vi "LinakUtilities.vi"(5 "LinakUtil":T1, 7 "Linak Address":u8=1, 8 "error in (no error)":errorcluster, 10 "Request(mm)":dbl=20.0 min=0.0 max=100000.0 step=10.0) -> (0 "error out":errorcluster, 1 "Target(mm)":dbl, 2 "AbsPosition":dbl, 3 "ThereYet?":bool)   [LabVIEW 2021]
uses:
  LINAKUTIL.ctl
  Registers.ctl
  <vilib>/Plasmionique/MB Master/MB_Master_TCP/MB_Master_TCP.lvclass
  Applications/National Instruments/LabVIEW 2021 64-bit/vi.lib/Plasmionique/MB Master/MB_Master/MB_Master.lvclass
  CPPSW/Systems/Cross-System/Fetch+RampsGlobal.vi
  <vilib>/Plasmionique/MB Master/MB Master.lvlib
  Applications/National Instruments/LabVIEW 2021 64-bit/vi.lib/Plasmionique/MB Master/MB_Master_TCP/MB_Master_TCP.lvclass
panel:
  in  "LINAK Gateway IP Address":string
  in  "Timeout (ms)":i32=500
  out "Request(pulses)":u16
  out "Target(pulses)":u16
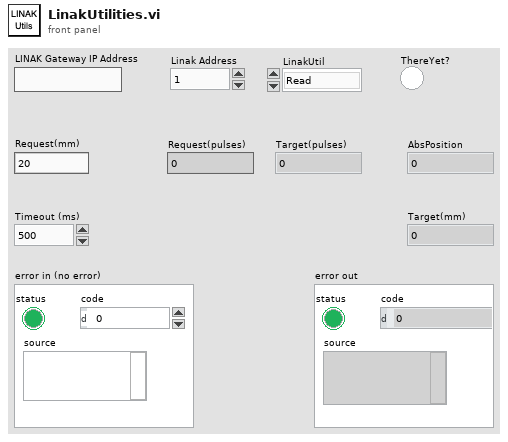
[diagram p1: front panel]
types:
  T1 = typedef "LINAKUTIL.ctl" = enum16{"Read", "ReadTarget", "WriteTarget", "SingleGo", "GlobalGo", "SafetySet", "WriteReadGo", "STOP"}
  T2 = typedef "Registers.ctl" = enum16{"Null", "TargetPosition", "Move"}
  T3 = typedef "LINAKStatusCluster.ctl" = cluster{"RunStatus":enum16{"Idle", "RunningOut", "RunningIn", "WaitingToRun", "InitOut", "InitIn"}, "ActualPosition(pulses)":u16, "DistanceFromTarget(pulses)":u16, "Status1":string, "ReasonForLastStop":string, "SupplyVoltage(V)":dbl, "Current(A)":dbl, "InternalTemp(C)":i16, "FETtemp(C)":i16}
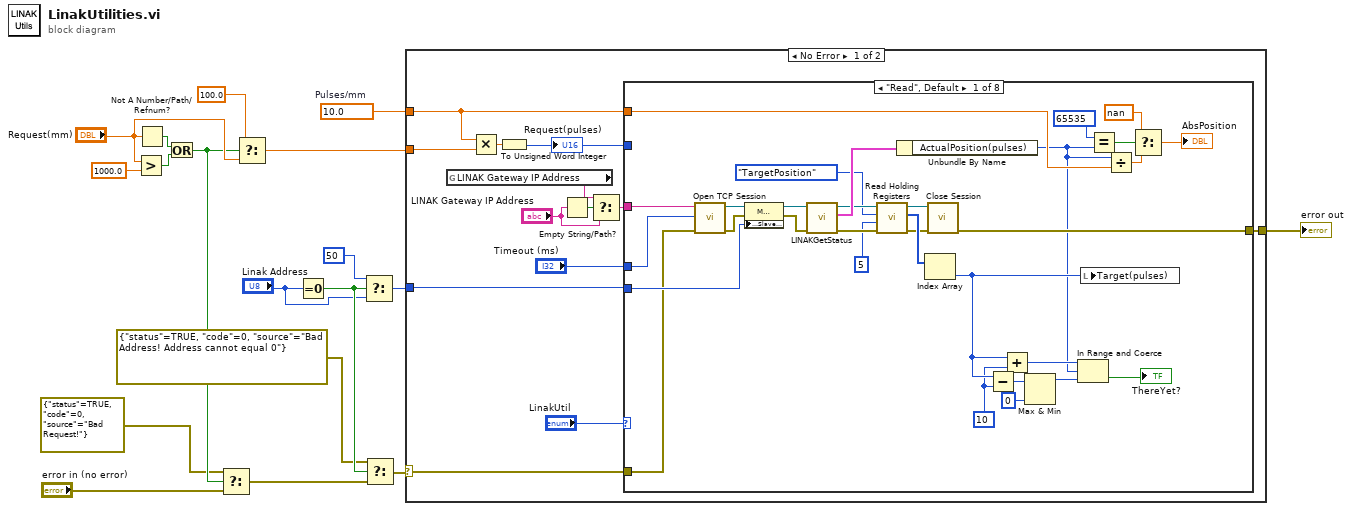
[diagram p0: block diagram]
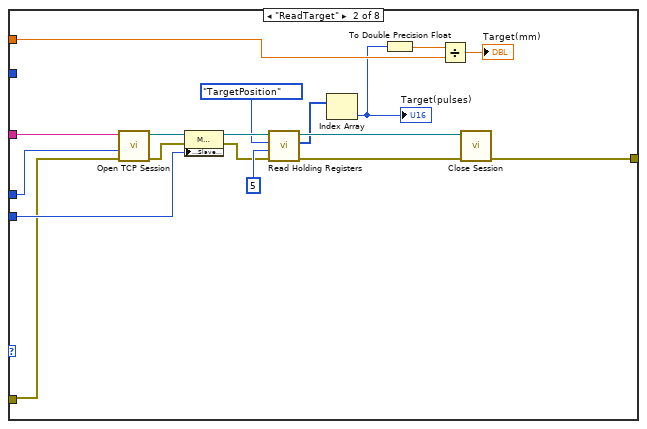
[diagram p2: hidden frame]
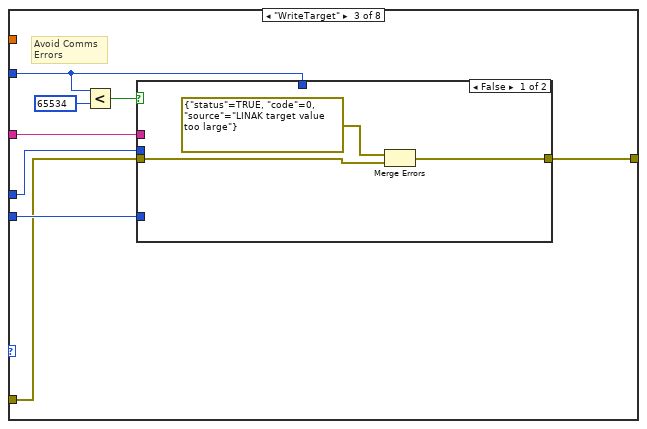
[diagram p3: hidden frame]
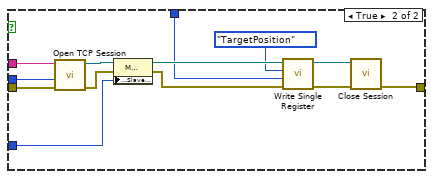
[diagram p4: hidden frame]
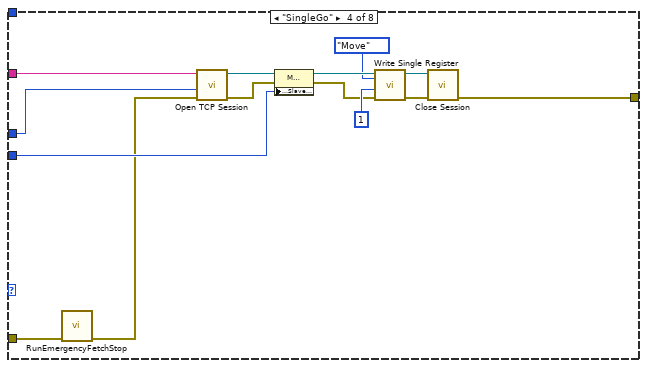
[diagram p5: hidden frame]
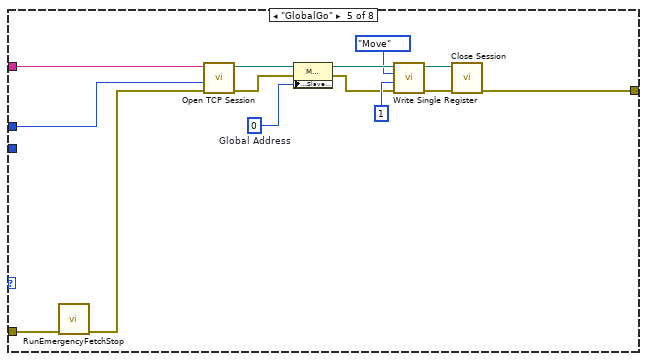
[diagram p6: hidden frame]
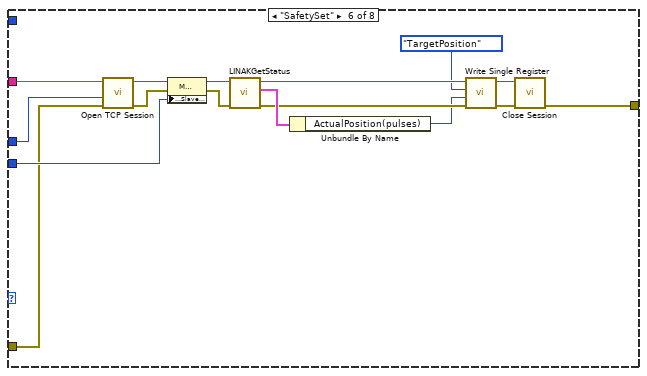
[diagram p7: hidden frame]
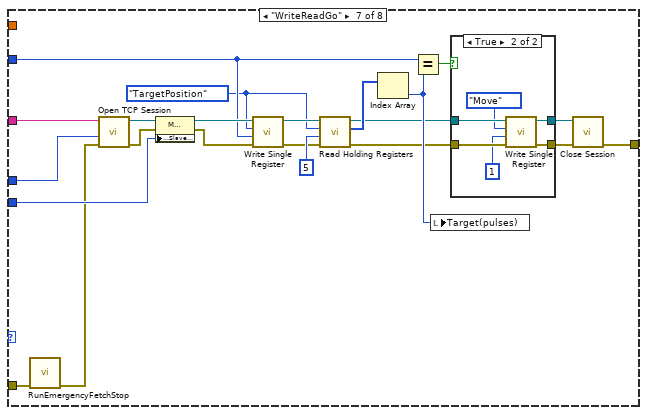
[diagram p8: hidden frame]
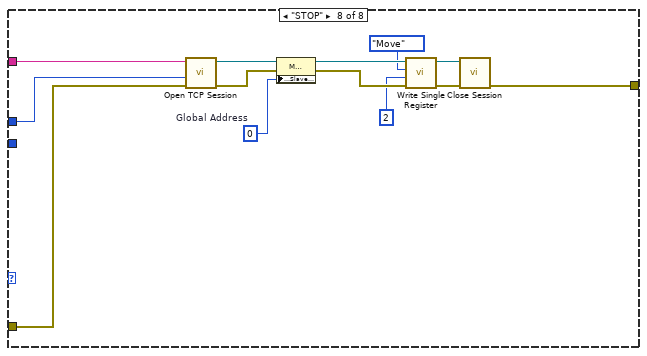
[diagram p10: hidden frame]
diagram:
  w1 = 10.0  # Pulses/mm
  n1 = Greater?(x="Request(mm)", y=1000.0) -> (0:w14:bool)
  n2 = Not A Number/Path/Refnum?(number/path/refnum="Request(mm)") -> (NaN/Path/Refnum?=w15:bool)
  n3 = Or(x=w15, y=w14) -> (x .or. y?=w9:bool)
  n4 = Select(t=errorcluster {"status"=TRUE, "code"=0, "source"="Bad Request!"}, s=w9, f="error in (no error)") -> (s? t:f=w6:errorcluster)
  n5 = Select(t=100.0, s=w9, f="Request(mm)") -> (s? t:f=w12:dbl)
  n6 = Equal To 0?(x="Linak Address") -> (x = 0?=w7:bool)
  n7 = Select(t=u8 50, s=w7, f="Linak Address") -> (s? t:f=w16:u8)
  n8 = Select(t=errorcluster {"status"=TRUE, "code"=0, "source"="Bad Address! Address cannot equal 0"}, s=w7, f=w6) -> (s? t:f=w4:errorcluster)
  n9 = case shown="No Error" w4 {
    selector: w4 -> [w20 w192]
    tunnel: [w28 w192] -> w18
    tunnel: w16 -> [w27 _]
    tunnel: w12 -> [w26 _]
    tunnel: w1 -> [w19 _]
    frame No Error {
      n10 = global read "Fetch+RampsGlobal.vi" "LINAK Gateway IP Address"() -> (w22:string)
      n11 = Multiply(x=w19, y=w26) -> (x*y=w31:dbl)
      n12 = To Unsigned Word Integer(number=w31) -> (unsigned 16bit integer=w30:u16)
      "Request(pulses)" <- w30
      n13 = Empty String/Path?(string/path="LINAK Gateway IP Address") -> (empty?=w24:bool)
      n14 = Select(t=w22, s=w24, f="LINAK Gateway IP Address") -> (s? t:f=w21:string)
      n15 = case shown="\"Read\", Default" "LinakUtil" {
        tunnel: w30 -> [_ _ w82 _ _ _ w161 _]
        tunnel: w19 -> [w61 w79 _ _ _ _ _ _]
        tunnel: w27 -> [w60 w80 w88 w118 _ w145 w170 _]
        tunnel: "Timeout (ms)" -> [w52 w73 w86 w116 w131 w143 w166 w184]
        tunnel: w21 -> [w51 w74 w87 w117 w132 w144 w167 w185]
        tunnel: w20 -> [w48 w72 w85 w106 w119 w142 w150 w183]
        tunnel: [w40 w65 w84 w115 w130 w135 w151 w190] -> w28
        frame "Read", Default {
          w53 = u16 10 ("y")
          n16 = call <vilib>:"Open TCP Session.vi"("error in (no error)"=w48, "Timeout (10000)"=w52, "IP Address"=w51) -> ("error out"=w49:errorcluster, "MB_TCP session"=w50:refnum<class "MB_Master_TCP.lvclass">)  [unwired: 7 in]
          n17 = property class="MB_Master_TCP"(reference=w50, error in=w49, "Properties:Slave ID"=w60) -> (reference out=w59:refnum<class "MB_Master_TCP.lvclass">, error out=w58:errorcluster)
          n18 = call "LINAKGetStatus.vi"("Error In"=w58, "MB_Master_TCP in"=w59) -> ("Error Out"=w46:errorcluster, "StatusCluster"=w62:T3, "MB_Master_TCP out"=w45:refnum<class "MB_Master_TCP.lvclass">)  [unwired: 7 in]
          n19 = call <vilib>:"Read Holding Registers.vi"("error in (no error)"=w46, "quantity"=u16 5 ("read quantity"), "starting address"=Registers."TargetPosition" ("LINAKregisters"), "MB session in"=w45) -> ("error out"=w41:errorcluster, "Registers"=w47:u16[], "MB session out"=w42:refnum<class "MB_Master_TCP.lvclass">)  [unwired: 5 in]
          n20 = Unbundle By Name(w62) -> ("ActualPosition(pulses)"=w34:u16)
          n21 = Index Array(array=w47) -> (element=w54:u16)  [unwired: 1 in]
          n22 = call-dynamic "Close Session.vi"("error in (no error)"=w41, "MB TCP session"=w42) -> ("error out"=w40:errorcluster)  [unwired: 9 in]
          n23 = Subtract(x=w54, y=w53) -> (x-y=w37:u16)
          n24 = Add(x=w54, y=w53) -> (x+y=w39:u16)
          n25 = Max & Min(x=w37, y=u16 0) -> (max(x,y)=w35:u16)  [unwired: 1 out]
          n26 = In Range and Coerce(upper limit=w39, x=w34, lower limit=w35) -> (In Range?=→"ThereYet?":bool)  [unwired: 1 out]
          n27 = local write "Target(pulses)"(w54) -> ()
          n28 = Equal?(x=u16 65535, y=w34) -> (x = y?=w32:bool)
          n29 = Divide(x=w34, y=w61) -> (x/y=w57:dbl)
          n30 = Select(t=nan, s=w32, f=w57) -> (s? t:f=→"AbsPosition":dbl)
        }
        frame "ReadTarget" {
          n31 = call <vilib>:"Open TCP Session.vi"("error in (no error)"=w72, "Timeout (10000)"=w73, "IP Address"=w74) -> ("error out"=w71:errorcluster, "MB_TCP session"=w75:refnum<class "MB_Master_TCP.lvclass">)  [unwired: 7 in]
          n32 = property class="MB_Master_TCP"(reference=w75, error in=w71, "Properties:Slave ID"=w80) -> (reference out=w70:refnum<class "MB_Master_TCP.lvclass">, error out=w67:errorcluster)
          n33 = call <vilib>:"Read Holding Registers.vi"("error in (no error)"=w67, "quantity"=u16 5 ("read quantity"), "starting address"=Registers."TargetPosition" ("LINAKregisters"), "MB session in"=w70) -> ("error out"=w66:errorcluster, "Registers"=w63:u16[], "MB session out"=w64:refnum<class "MB_Master_TCP.lvclass">)  [unwired: 5 in]
          n34 = Index Array(array=w63) -> (element=w78:u16)  [unwired: 1 in]
          "Target(pulses)" <- w78
          n35 = To Double Precision Float(number=w78) -> (double precision float=w77:dbl)
          n36 = Divide(x=w77, y=w79) -> (x/y=→"Target(mm)":dbl)
          n37 = call-dynamic "Close Session.vi"("error in (no error)"=w66, "MB TCP session"=w64) -> ("error out"=w65:errorcluster)  [unwired: 9 in]
        }
        frame "WriteTarget" {
          # "Avoid Comms\nErrors"
          n38 = Less?(x=w82, y=u16 65534) -> (x < y?=w83:bool)
          n39 = case shown="False" w83 {
            tunnel: w82 -> [_ w95]
            tunnel: w88 -> [_ w104]
            tunnel: w87 -> [_ w103]
            tunnel: w86 -> [_ w102]
            tunnel: w85 -> [w89 w101]
            tunnel: [w90 w92] -> w84
            frame False {
              n40 = Merge Errors(errorcluster {"status"=TRUE, "code"=0, "source"="LINAK target value too large"} ("error in"), w89) -> (w90:errorcluster)
            }
            frame True {
              n41 = call <vilib>:"Open TCP Session.vi"("error in (no error)"=w101, "Timeout (10000)"=w102, "IP Address"=w103) -> ("error out"=w100:errorcluster, "MB_TCP session"=w99:refnum<class "MB_Master_TCP.lvclass">)  [unwired: 7 in]
              n42 = property class="MB_Master_TCP"(reference=w99, error in=w100, "Properties:Slave ID"=w104) -> (reference out=w97:refnum<class "MB_Master_TCP.lvclass">, error out=w98:errorcluster)
              n43 = call <vilib>:"Write Single Register.vi"("error in (no error)"=w98, "value"=w95, "address"=Registers."TargetPosition" ("LINAKregisters"), "MB session in"=w97) -> ("error out"=w93:errorcluster, "MB session out"=w94:refnum<class "MB_Master_TCP.lvclass">)  [unwired: 6 in]
              n44 = call-dynamic "Close Session.vi"("error in (no error)"=w93, "MB TCP session"=w94) -> ("error out"=w92:errorcluster)  [unwired: 9 in]
            }
          }
        }
        frame "SingleGo" {
          n45 = call "RunEmergencyFetchStop.vi"("error in (no error)"=w106) -> ("error out"=w105:errorcluster)  [unwired: 6 in]
          n46 = call <vilib>:"Open TCP Session.vi"("error in (no error)"=w105, "Timeout (10000)"=w116, "IP Address"=w117) -> ("error out"=w114:errorcluster, "MB_TCP session"=w113:refnum<class "MB_Master_TCP.lvclass">)  [unwired: 7 in]
          n47 = property class="MB_Master_TCP"(reference=w113, error in=w114, "Properties:Slave ID"=w118) -> (reference out=w112:refnum<class "MB_Master_TCP.lvclass">, error out=w109:errorcluster)
          n48 = call <vilib>:"Write Single Register.vi"("error in (no error)"=w109, "value"=u16 1, "address"=Registers."Move" ("LINAKregisters"), "MB session in"=w112) -> ("error out"=w108:errorcluster, "MB session out"=w107:refnum<class "MB_Master_TCP.lvclass">)  [unwired: 6 in]
          n49 = call-dynamic "Close Session.vi"("error in (no error)"=w108, "MB TCP session"=w107) -> ("error out"=w115:errorcluster)  [unwired: 9 in]
        }
        frame "GlobalGo" {
          w129 = u8 0  # Global Address
          n50 = call "RunEmergencyFetchStop.vi"("error in (no error)"=w119) -> ("error out"=w120:errorcluster)  [unwired: 6 in]
          n51 = call <vilib>:"Open TCP Session.vi"("error in (no error)"=w120, "Timeout (10000)"=w131, "IP Address"=w132) -> ("error out"=w128:errorcluster, "MB_TCP session"=w127:refnum<class "MB_Master_TCP.lvclass">)  [unwired: 7 in]
          n52 = property class="MB_Master_TCP"(reference=w127, error in=w128, "Properties:Slave ID"=w129) -> (reference out=w126:refnum<class "MB_Master_TCP.lvclass">, error out=w123:errorcluster)
          n53 = call <vilib>:"Write Single Register.vi"("error in (no error)"=w123, "value"=u16 1, "address"=Registers."Move" ("LINAKregisters"), "MB session in"=w126) -> ("error out"=w122:errorcluster, "MB session out"=w121:refnum<class "MB_Master_TCP.lvclass">)  [unwired: 6 in]
          n54 = call-dynamic "Close Session.vi"("error in (no error)"=w122, "MB TCP session"=w121) -> ("error out"=w130:errorcluster)  [unwired: 9 in]
        }
        frame "SafetySet" {
          n55 = call <vilib>:"Open TCP Session.vi"("error in (no error)"=w142, "Timeout (10000)"=w143, "IP Address"=w144) -> ("error out"=w140:errorcluster, "MB_TCP session"=w141:refnum<class "MB_Master_TCP.lvclass">)  [unwired: 7 in]
          n56 = property class="MB_Master_TCP"(reference=w141, error in=w140, "Properties:Slave ID"=w145) -> (reference out=w147:refnum<class "MB_Master_TCP.lvclass">, error out=w148:errorcluster)
          n57 = call "LINAKGetStatus.vi"("Error In"=w148, "MB_Master_TCP in"=w147) -> ("Error Out"=w134:errorcluster, "StatusCluster"=w146:T3, "MB_Master_TCP out"=w139:refnum<class "MB_Master_TCP.lvclass">)  [unwired: 7 in]
          n58 = Unbundle By Name(w146) -> ("ActualPosition(pulses)"=w133:u16)
          n59 = call <vilib>:"Write Single Register.vi"("error in (no error)"=w134, "value"=w133, "address"=Registers."TargetPosition" ("LINAKregisters"), "MB session in"=w139) -> ("error out"=w136:errorcluster, "MB session out"=w137:refnum<class "MB_Master_TCP.lvclass">)  [unwired: 6 in]
          n60 = call-dynamic "Close Session.vi"("error in (no error)"=w136, "MB TCP session"=w137) -> ("error out"=w135:errorcluster)  [unwired: 9 in]
        }
        frame "WriteReadGo" {
          w159 = Registers."TargetPosition" ("LINAKregisters")
          n61 = call "RunEmergencyFetchStop.vi"("error in (no error)"=w150) -> ("error out"=w149:errorcluster)  [unwired: 6 in]
          n62 = call <vilib>:"Open TCP Session.vi"("error in (no error)"=w149, "Timeout (10000)"=w166, "IP Address"=w167) -> ("error out"=w165:errorcluster, "MB_TCP session"=w164:refnum<class "MB_Master_TCP.lvclass">)  [unwired: 7 in]
          n63 = property class="MB_Master_TCP"(reference=w164, error in=w165, "Properties:Slave ID"=w170) -> (reference out=w163:refnum<class "MB_Master_TCP.lvclass">, error out=w160:errorcluster)
          n64 = call <vilib>:"Write Single Register.vi"("error in (no error)"=w160, "value"=w161, "address"=w159, "MB session in"=w163) -> ("error out"=w157:errorcluster, "MB session out"=w162:refnum<class "MB_Master_TCP.lvclass">)  [unwired: 6 in]
          n65 = call <vilib>:"Read Holding Registers.vi"("error in (no error)"=w157, "quantity"=u16 5 ("read quantity"), "starting address"=w159, "MB session in"=w162) -> ("error out"=w155:errorcluster, "Registers"=w156:u16[], "MB session out"=w154:refnum<class "MB_Master_TCP.lvclass">)  [unwired: 5 in]
          n66 = Index Array(array=w156) -> (element=w169:u16)  [unwired: 1 in]
          n67 = Equal?(x=w161, y=w169) -> (x = y?=w168:bool)
          n68 = local write "Target(pulses)"(w169) -> ()
          n69 = case shown="True" w168 {
            tunnel: w154 -> [w171 w178]
            tunnel: w155 -> [w172 w175]
            tunnel: [w171 w177] -> w153
            tunnel: [w172 w176] -> w152
            frame False {
            }
            frame True {
              n70 = call <vilib>:"Write Single Register.vi"("error in (no error)"=w175, "value"=u16 1, "address"=Registers."Move" ("LINAKregisters"), "MB session in"=w178) -> ("error out"=w176:errorcluster, "MB session out"=w177:refnum<class "MB_Master_TCP.lvclass">)  [unwired: 6 in]
            }
          }
          n71 = call-dynamic "Close Session.vi"("error in (no error)"=w152, "MB TCP session"=w153) -> ("error out"=w151:errorcluster)  [unwired: 9 in]
        }
        frame "STOP" {
          w191 = u8 0  # Global Address
          n72 = call <vilib>:"Open TCP Session.vi"("error in (no error)"=w183, "Timeout (10000)"=w184, "IP Address"=w185) -> ("error out"=w182:errorcluster, "MB_TCP session"=w186:refnum<class "MB_Master_TCP.lvclass">)  [unwired: 7 in]
          n73 = property class="MB_Master_TCP"(reference=w186, error in=w182, "Properties:Slave ID"=w191) -> (reference out=w187:refnum<class "MB_Master_TCP.lvclass">, error out=w181:errorcluster)
          n74 = call <vilib>:"Write Single Register.vi"("error in (no error)"=w181, "value"=u16 2, "address"=Registers."Move" ("LINAKregisters"), "MB session in"=w187) -> ("error out"=w188:errorcluster, "MB session out"=w189:refnum<class "MB_Master_TCP.lvclass">)  [unwired: 6 in]
          n75 = call-dynamic "Close Session.vi"("error in (no error)"=w188, "MB TCP session"=w189) -> ("error out"=w190:errorcluster)  [unwired: 9 in]
        }
      }
    }
    frame Error {
    }
  }
  "error out" <- w18
